vi "Post-Build Custom Action.vi"(10 "Variant":variant) -> (0 "error out":errorcluster)   [LabVIEW 2016]
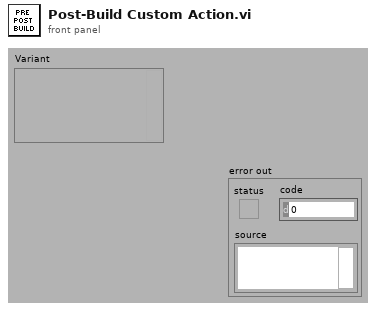
[diagram p1: front panel]
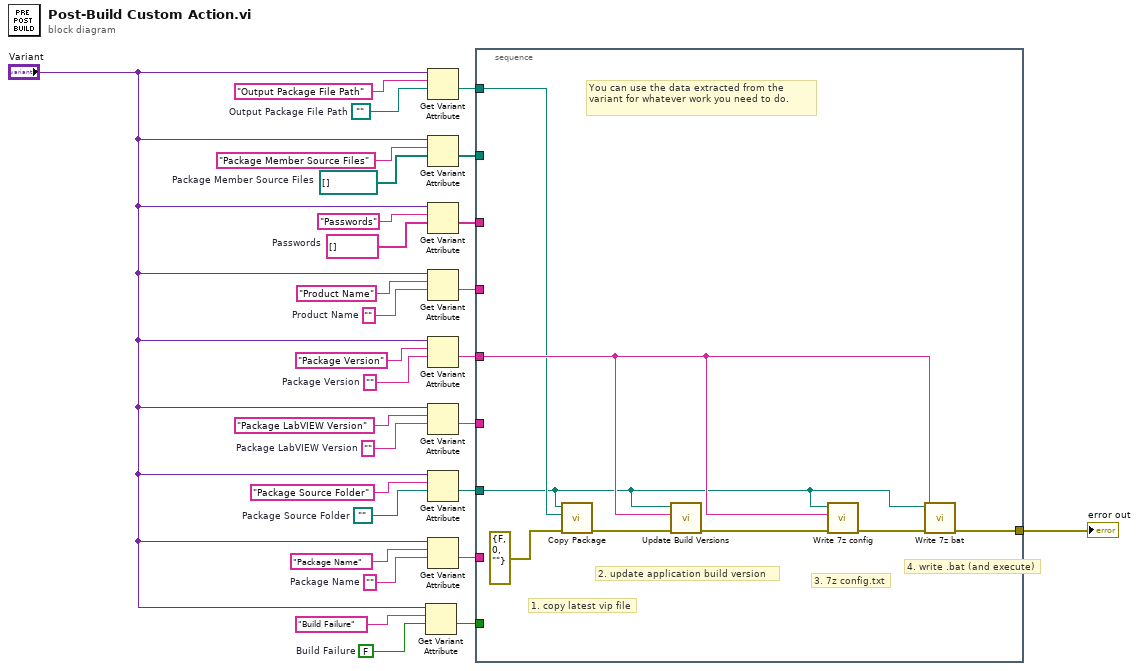
[diagram p0: block diagram]
diagram:
  w4 = FALSE  # Build Failure
  w14 = path ""  # Package Source Folder
  w15 = ""  # Package Name
  w18 = ""  # Package LabVIEW Version
  w20 = ""  # Package Version
  w22 = ""  # Product Name
  w24 = string[] []  # Passwords
  w26 = path[] []  # Package Member Source Files
  w28 = path ""  # Output Package File Path
  n1 = Get Variant Attribute(Variant="Variant", name="Build Failure", default value (empty Variant)=w4) -> (value=w2:bool)  [unwired: 1 in, 3 out]
  n2 = Get Variant Attribute(Variant="Variant", name="Output Package File Path", default value (empty Variant)=w28) -> (value=w13:path)  [unwired: 1 in, 3 out]
  n3 = Get Variant Attribute(Variant="Variant", name="Package Member Source Files", default value (empty Variant)=w26) -> (value=w12:path[])  [unwired: 1 in, 3 out]
  n4 = Get Variant Attribute(Variant="Variant", name="Passwords", default value (empty Variant)=w24) -> (value=w11:string[])  [unwired: 1 in, 3 out]
  n5 = Get Variant Attribute(Variant="Variant", name="Product Name", default value (empty Variant)=w22) -> (value=w10:string)  [unwired: 1 in, 3 out]
  n6 = Get Variant Attribute(Variant="Variant", name="Package Version", default value (empty Variant)=w20) -> (value=w9:string)  [unwired: 1 in, 3 out]
  n7 = Get Variant Attribute(Variant="Variant", name="Package LabVIEW Version", default value (empty Variant)=w18) -> (value=w8:string)  [unwired: 1 in, 3 out]
  n8 = Get Variant Attribute(Variant="Variant", name="Package Source Folder", default value (empty Variant)=w14) -> (value=w7:path)  [unwired: 1 in, 3 out]
  n9 = Get Variant Attribute(Variant="Variant", name="Package Name", default value (empty Variant)=w15) -> (value=w6:string)  [unwired: 1 in, 3 out]
  n10 = stacked-sequence {
    tunnel: w13 -> [w31]
    tunnel: w12 -> [_]
    tunnel: w11 -> [_]
    tunnel: w10 -> [_]
    tunnel: w9 -> [w34]
    tunnel: w8 -> [_]
    tunnel: w7 -> [w30]
    tunnel: w6 -> [_]
    tunnel: w2 -> [_]
    tunnel: [w37] -> w1
    frame #0 {
      # "2. update application build version"
      # "1. copy latest vip file"
      # "3. 7z config.txt"
      # "4. write .bat (and execute)"
      # "You can use the data extracted from the variant for whatever work you need to do."
      n11 = call "Copy Package.vi"("error in (no error)"=errorcluster {"status"=FALSE, "code"=0, "source"=""} ("error in"), "Output Package File Path"=w31, "Package Source Folder"=w30) -> ("error out"=w33:errorcluster)  [unwired: 8 in]
      n12 = call "Update Build Versions.vi"("error in (no error)"=w33, "Package Version"=w34, "Package Source Folder"=w30) -> ("error out"=w35:errorcluster)  [unwired: 8 in]
      n13 = call "Write 7z config.vi"("error in (no error)"=w35, "Package Version"=w34, "Package Source Folder"=w30) -> ("error out"=w36:errorcluster)  [unwired: 8 in]
      n14 = call "Write 7z bat.vi"("error in (no error)"=w36, "Package Version"=w34, "source path"=w30) -> ("error out"=w37:errorcluster)  [unwired: 8 in]
    }
  }
  "error out" <- w1
